vi "Close Connection.vi"(8 "error in (no error)":errorcluster, 11 "RemoteControl in":refnum<class "RemoteControl.lvclass">) -> (0 "error out":errorcluster, 3 "RemoteControl out":refnum<class "RemoteControl.lvclass">)   [LabVIEW 2019, in "RemoteControl.lvlib" / "RemoteControl.lvclass"]
uses:
  RemoteControl.lvclass
  Typedefs/Message--Cluster.ctl
  RemoteControl.lvclass/RemoteControl.ctl
  Private/RemoteControl.GlobalVariable.vi
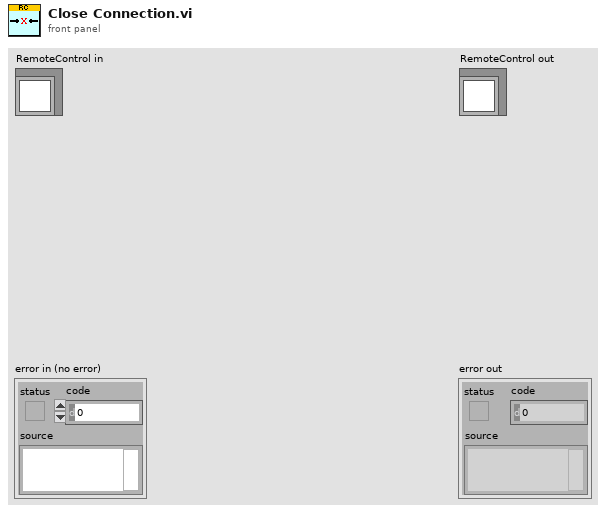
[diagram p1: front panel]
types:
  T1 = typedef "RemoteControl.lvlib/RemoteControl.lvclass/Message--Cluster.ctl" = cluster{"Command":string, "Data":variant, "ID":string}
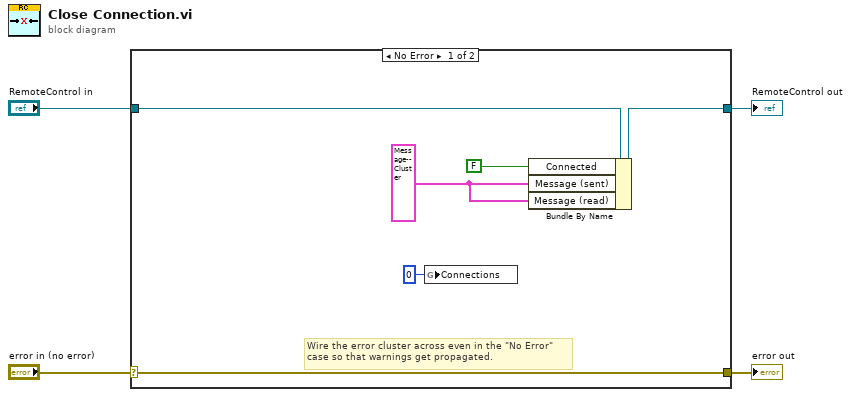
[diagram p0: block diagram]
diagram:
  n1 = case shown="No Error" "error in (no error)" {
    selector: "error in (no error)" -> [w10 w12]
    tunnel: [w10 w12] -> w1
    tunnel: [w8 w11] -> w2
    tunnel: "RemoteControl in" -> [w9 w11]
    frame No Error {
      w6 = T1 {"Command"="", "Data"=variant(string ""), "ID"=""} ("Message (sent)")
      # "Wire the error cluster across even in the \"No Error\"\ncase so that warnings get propagated."
      n2 = global write "RemoteControl.GlobalVariable.vi" "Connections"(0 ("Connections")) -> ()
      n3 = Bundle By Name(cluster=w9, "Connected"=FALSE ("Created"), "Message (sent)"=w6, "Message (read)"=w6) -> (w8:refnum<class "RemoteControl.lvclass">)
    }
    frame Error {
    }
  }
  "error out" <- w1
  "RemoteControl out" <- w2
